vi "Create Data Channel - Array - Type Cast.vi"(8 "error in (no error)":errorcluster, 9 "settings":T2, 10 "channel name":string, 11 "response refnum in":T1 format="%.0x") -> (0 "error out":errorcluster, 2 "channel refnums":T1[](array[typedef]) format="%.0x", 3 "response refnum out":T1 format="%.0x")   [LabVIEW 2018, in "Instrument Addon Scripting API.lvlib"]
doc: "Creates a new Data Channel with the following configuration:\nData Type: Array\nChannel Type: Type Cast\n\nIt also creates all the channel elements specified in the \"Elements\" array from the \"Settings\" input.\n\nInput: \nMessage Refnum In: reference to the \"Response\" message section.\nName: represents the desired name of the Data Channel.\nSettings: represents the settings applied as well as the settings for each element which will be added to the Data Channel.\n\nOutput:\nMessage Refnum Out: reference to the \"Response\" message section used as input.\nChannel Refnums: reference to the newly created Data Channels."
uses:
  Instrument Addon Scripting API.lvlib
  <vilib>/NI Veristand/Custom Device API/Custom Device Item Ref.ctl
  TypeDefs/Array Type Cast Settings.ctl
  TypeDefs/Array Element.ctl
  Addon/Addon Shared/Types/Type Cast Type.ctl
  Addon/Addon Shared/Types/Endian.ctl
  Addon/Addon Shared/Types/Data Parameters.ctl
  Addon/Addon Shared/Types/Protocol Data Type.ctl
  Addon/Addon Shared/Types/Data Channel Type.ctl
  Addon/Addon Shared/Instrument Addon Shared.lvlib
  <vilib>/NI Veristand/Custom Device API/Custom Device API.lvlib
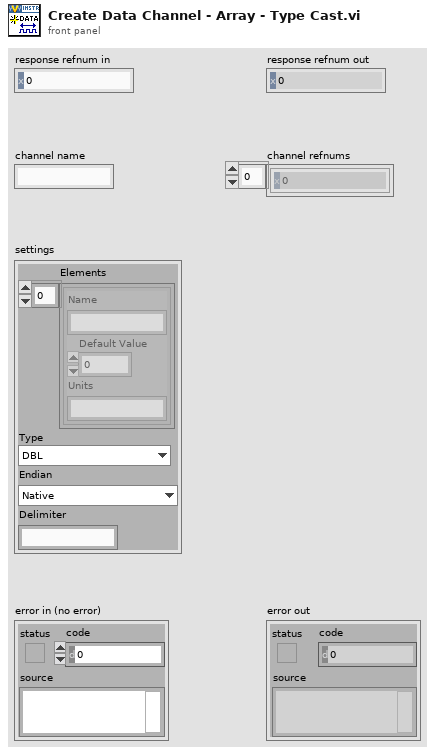
[diagram p1: front panel]
types:
  T1 = typedef "Custom Device API.lvlib/Custom Device Item Ref.ctl" = u64
  T2 = typedef "Instrument Addon Scripting API.lvlib/Array Type Cast Settings.ctl" = cluster{"Elements":T3[], "Type":T4, "Endian":T5, "Delimiter":string}
  T3 = typedef "Instrument Addon Scripting API.lvlib/Array Element.ctl" = cluster{"Name":string, "Default Value":dbl, "Units":string}
  T4 = typedef "Instrument Addon Shared.lvlib/Type Cast Type.ctl" = enum16{"DBL", "SGL", "U64", "U32", "U16", "U8", "I64", "I32", "I16", "I8"}
  T5 = typedef "Instrument Addon Shared.lvlib/Endian.ctl" = enum16{"Native", "Little", "Big"}
  T6 = typedef "Instrument Addon Shared.lvlib/Data Channel Type.ctl" = enum16{"Format", "Comparison", "Type Cast", "Enumerated List"}
  T7 = typedef "Instrument Addon Shared.lvlib/Protocol Data Type.ctl" = enum16{"Single Channel", "Array"}
  T8 = typedef "Instrument Addon Shared.lvlib/Data Parameters.ctl" = cluster{"Data Type":T7, "Channel Type":T6, "Format String":string, "Expected String":string, "Type":T4, "List":string[], "Delimiter":string, "Endian":T5}
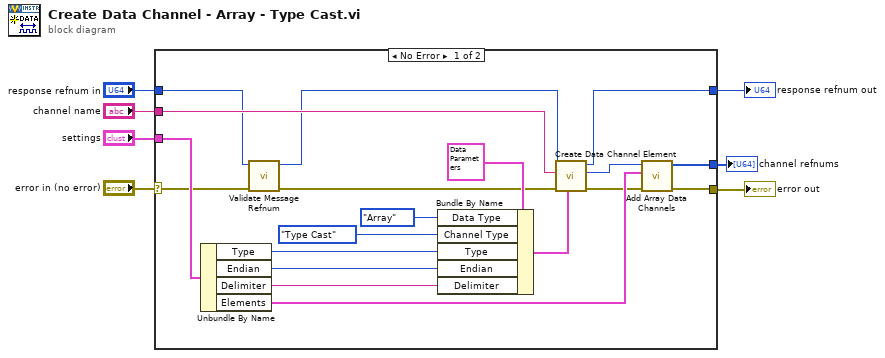
[diagram p0: block diagram]
diagram:
  n1 = case shown="No Error" "error in (no error)" {
    selector: "error in (no error)" -> [w11 w28]
    tunnel: [w21 w28] -> w7
    tunnel: [w14 w27] -> w6
    tunnel: "channel name" -> [w16 _]
    tunnel: "response refnum in" -> [w10 w27]
    tunnel: "settings" -> [w20 _]
    tunnel: [w19 _] -> w1
    frame No Error {
      n2 = Unbundle By Name(w20) -> ("Type"=w23:T4, "Endian"=w22:T5, "Delimiter"=w17:string, "Elements"=w18:T3[])
      n3 = call "Validate Message Refnum.vi"("error in (no error)"=w11, "Message in"=w10) -> ("error out"=w8:errorcluster, "Message out"=w9:T1)  [unwired: 8 in]
      n4 = Bundle By Name(cluster=T8 {"Data Type"=enum."Array", "Channel Type"=enum."Format", "Format String"="%.3g", "Expected String"="", "Type"=enum."SGL", "List"=[], "Delimiter"=",", "Endian"=enum."Native"} ("Settings"), "Data Type"=Protocol_Data_Type."Array", "Channel Type"=Data_Channel_Type."Type Cast", "Type"=w23, "Endian"=w22, "Delimiter"=w17) -> (w15:T8)
      n5 = call "Create Data Channel Element.vi"("Data Channel Parameters"=w15, "Error In"=w8, "Name"=w16, "Refnum In"=w9) -> ("Error Out"=w12:errorcluster, "Channel Refnum"=w13:T1, "Refnum Out"=w14:T1)  [unwired: 5 in]
      n6 = call "Add Array Data Channels.vi"("Error In"=w12, "Array Elements"=w18, "Section Refnum In"=w13) -> ("Error Out"=w21:errorcluster, "Channel Refnums"=w19:T1[])  [unwired: 7 in]
    }
    frame Error {
    }
  }
  "error out" <- w7
  "response refnum out" <- w6
  "channel refnums" <- w1
